vi "c_ctre_phoenix6_deserialize_pgn.vi"(0 "Numeric 2":i32, 1 "String 2":string, 2 "Numeric 3":u32, 3 "Numeric 5":u16, 4 "Numeric 7":u16) -> (20 "Numeric":i32, 21 "String":string, 22 "Numeric 4":u16, 23 "Numeric 6":u16)   [LabVIEW 2023]
uses:
  <vilib>/Rock Robotics/WPI/ThirdParty/Phoenix-LabVIEW/Controls/DriverLib.ctl
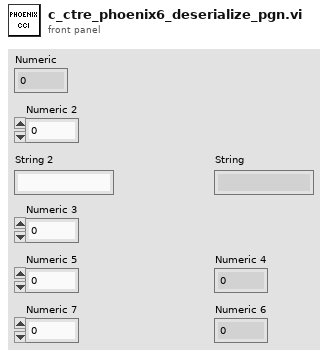
[diagram p1: front panel]
types:
  T1 = typedef "DriverLib.ctl" = path
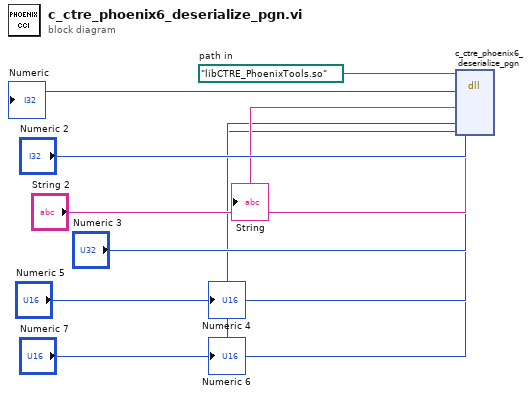
[diagram p0: block diagram]
diagram:
  w10 = T1 path "libCTRE_PhoenixTools.so"  # path in
  n1 = dll-call lib="?" fn="c_ctre_phoenix6_deserialize_pgn"(path in=w10, "Numeric 2", "String 2", "Numeric 3", "Numeric 5", "Numeric 7") -> (→"Numeric":i32, →"String":string, →"Numeric 4":u16, →"Numeric 6":u16)  [unwired: 4 in, 2 out]
